vi "frontp_stop_all_subpanels.vi"(8 "error in (no error)":errorcluster, 11 "front_panel in":refnum<class "front_panel.lvclass">) -> (0 "error out":errorcluster, 3 "front_panel out":refnum<class "front_panel.lvclass">)   [LabVIEW 2015, in "front_panel.lvclass"]
uses:
  front_panel.lvclass
  front_panel.lvclass/front_panel.ctl
  <vilib>/ActorFramework/Message Enqueuer/Message Enqueuer.lvclass/Message Enqueuer.ctl
  <vilib>/ActorFramework/Message Enqueuer/Enqueue.vi
  <vilib>/ActorFramework/Message Priority Queue/Priority Enqueue.vi
  <vilib>/ActorFramework/Stop Msg/Stop Msg.lvclass
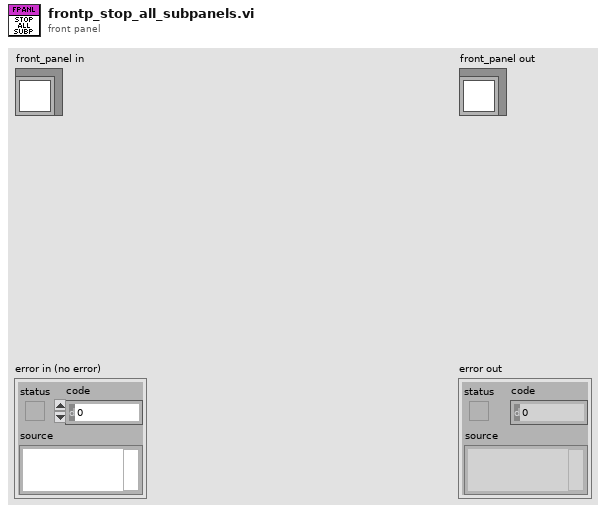
[diagram p1: front panel]
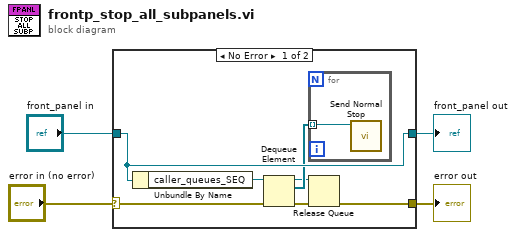
[diagram p0: block diagram]
diagram:
  n1 = case shown="No Error" "error in (no error)" {
    selector: "error in (no error)" -> [w9 w14]
    tunnel: [w5 w14] -> w3
    tunnel: [w11 w13] -> w1
    tunnel: "front_panel in" -> [w11 w13]
    frame No Error {
      n2 = Unbundle By Name(w11) -> ("caller_queues_SEQ"=w10:refnum<queue>)
      n3 = Dequeue Element(queue=w10, error in (no error)=w9) -> (queue out=w6:refnum<queue>, element=w8:refnum<class "Message Enqueuer.lvclass">[], error out=w7:errorcluster)  [unwired: 1 in, 1 out]
      n4 = for {
        tunnel: w8 -> [w12] mode=indexing
        n5 = call <vilib>:"Send Normal Stop.vi"("Message Enqueuer"=w12) -> ()  [unwired: 10 in, 1 out]
      }
      n6 = Release Queue(queue=w6, error in (no error)=w7) -> (error out=w5:errorcluster)  [unwired: 1 in, 2 out]
    }
    frame Error {
    }
  }
  "error out" <- w3
  "front_panel out" <- w1
